vi "Config_calibr_04_03_2020.vi"(8 "error in (no error)":errorcluster, 10 "Acq parameters":T2 {"Frecuencia de muestreo y módulo CRIO" items=["51.200 kS/s (NI 9234)"=1, "25.600 kS/s (NI 9234)"=2, "17.067 kS/s (NI 9234)"=3, "12.800 kS/s (NI 9234)"=4, "10.240 kS/s (NI 9234)"=5, "8.533 kS/s (NI 9234)"=6, "7.314 kS/s (NI 9234)"=7, "6.400 kS/s (NI 9234)"=8, "5.689 kS/s (NI 9234)"=9, "5.120 kS/s (NI 9234)"=10, "4.654 kS/s (NI 9234)"=11, "4.267 kS/s (NI 9234)"=12, "3.938 kS/s (NI 9234)"=13, "3.657 kS/s (NI 9234)"=14, "3.413 kS/s (NI 9234)"=15, "3.200 kS/s (NI 9234)"=16, "3.012 kS/s (NI 9234)"=17, "2.845 kS/s (NI 9234)"=18, "2.695 kS/s (NI 9234)"=19, "2.560 kS/s (NI 9234)"=20, "2.438 kS/s (NI 9234)"=21, "2.328 kS/s (NI 9234)"=22, "2.226 kS/s (NI 9234)"=23, "2.133 kS/s (NI 9234)"=24, "2.048 kS/s (NI 9234)"=25, "1.969 kS/s (NI 9234)"=26, "1.896 kS/s (NI 9234)"=27, "1.829 kS/s (NI 9234)"=28, "1.765 kS/s (NI 9234)"=29, "1.707 kS/s (NI 9234)"=30, "1.652 kS/s (NI 9234)"=31]}, 11 "Refnum in":refnum<k20>) -> (0 "error out":errorcluster, 1 "Block Size":u32, 2 "Time to Acquire Block (ms)":i32, 3 "Refnum out":refnum<k20>)   [LabVIEW 2015]
uses:
  <vilib>/LabVIEW Targets/FPGA/cRIO/shared/nicrio_ModuleControls/nicrio_cRIO-9234_DataRatesRing2.ctl
  <vilib>/Utility/error.llb/Error Cluster From Error Code.vi
  <vilib>/rvi/errors/niLvFpgaAdjustHostInterfaceError.vi
  <vilib>/rvi/interface/common/niFpgaWaitOnOcc.vi
  <vilib>/rvi/interface/nirviReadWriteControl/nirviReadWriteControl.xnode
  FPGA Bitfiles/W&RDArabia_FPGATarget_FPGA8a2wsBIdirec_yJvL9yuTbZw.lvbitx
  <vilib>/rvi/interface/nirviMethod/nirviMethod.xnode
  <vilib>/FPGAPlugInAG/cRIO-9031/niLvFpga_ConfigureFifo_cRIO-9031.vi
  <vilib>/rvi/errors/niLvFpgaMergeErrorWithErrorCode.vi
  <vilib>/FPGAPlugInAG/cRIO-9031/niLvFpga_StartFifo_cRIO-9031.vi
  NiFpgaLv.dll
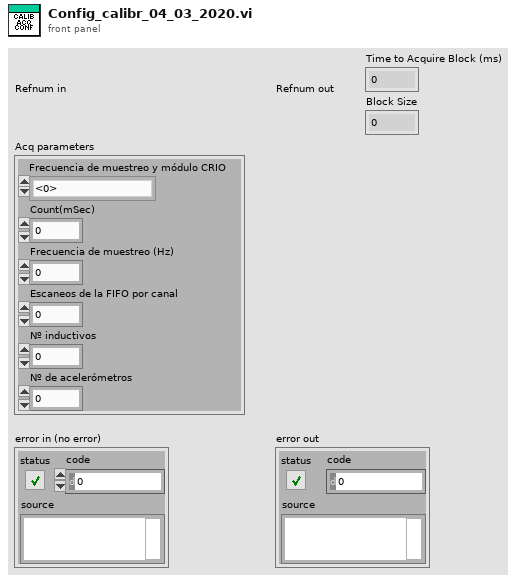
[diagram p1: front panel]
types:
  T1 = typedef "nicrio_cRIO-9234_DataRatesRing2.ctl" = u8
  T2 = cluster{"Frecuencia de muestreo y módulo CRIO":T1, "Count(mSec)":u32, "Frecuencia de muestreo (Hz)":dbl, "Escaneos de la FIFO por canal":u32, "Nº inductivos":i32, "Nº de acelerómetros":i32}
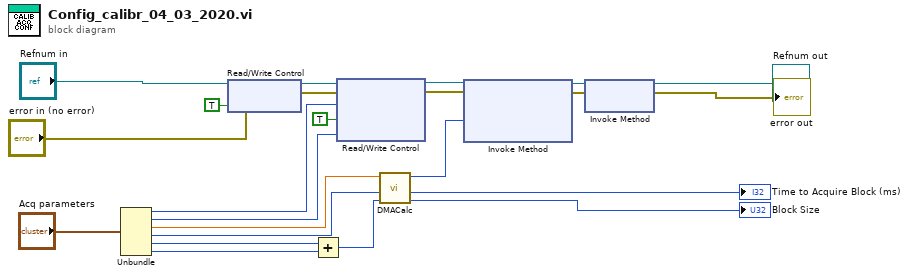
[diagram p0: block diagram]
diagram:
  n1 = Unbundle("Acq parameters") -> ("Frecuencia de muestreo y módulo CRIO"=w18:T1, "Count(mSec)"=w19:u32, "Frecuencia de muestreo (Hz)"=w20:dbl, "Escaneos de la FIFO por canal"=w21:u32, "Nº inductivos"=w22:i32, "Nº de acelerómetros"=w23:i32)
  n2 = xnode "Read/Write Control"("FPGA VI Reference In"="Refnum in", "error in"="error in (no error)", "Fotocélula"=TRUE ("Adquirir")) -> ("FPGA VI Reference Out"=w7:refnum<k20>, "error out"=w6:errorcluster)
  n3 = Add(x=w22, y=w23) -> (x+y=w3:i32)
  n4 = xnode "Read/Write Control"("FPGA VI Reference In"=w7, "error in"=w6, "Data Rate"=w18, "Digital?"=TRUE, "Count(mSec)"=w19) -> ("FPGA VI Reference Out"=w9:refnum<k20>, "error out"=w8:errorcluster)
  n5 = call "DMACalc.vi"("Number of Channels"=w3, "Number of Samples"=w21, "Rate (Hz)"=w20) -> ("Block Size"=→"Block Size":u32, "Time to Acquire Block (ms)"=→"Time to Acquire Block (ms)":i32, "Host Buffer Size"=w10:u32)  [unwired: 6 in]
  n6 = xnode "Invoke Method"("FPGA VI Reference In"=w9, "error in"=w8, "Requested Depth"=w10) -> ("FPGA VI Reference Out"=w12:refnum<k20>, "error out"=w11:errorcluster)  [unwired: 1 out]
  n7 = xnode "Invoke Method"("FPGA VI Reference In"=w12, "error in"=w11) -> ("FPGA VI Reference Out"=→"Refnum out":refnum<k20>, "error out"=→"error out":errorcluster)
